vi "Demo - Generate Analog Out Data.vi"(9 "Phase Offset (Radians)":dbl[](array[numeric]), 10 "Number of Samples":i32, 11 "Number of AO Channels":i32) -> (3 "Sine Wave":i16[][](array[numeric]))   [LabVIEW 2017]
doc: "Generates a set of sine waves, with a phase offset."
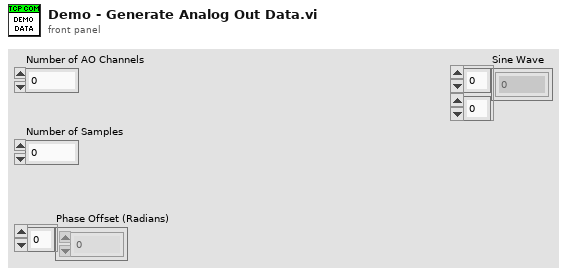
[diagram p1: front panel]
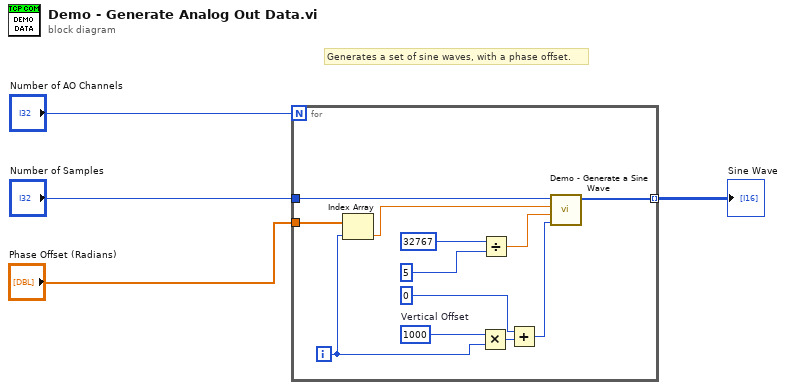
[diagram p0: block diagram]
diagram:
  # "Generates a set of sine waves, with a phase offset."
  n1 = for {
    N: "Number of AO Channels" -> [_]
    tunnel: "Number of Samples" -> [w13]
    tunnel: [w11] -> w4 mode=indexing
    tunnel: "Phase Offset (Radians)" -> [w10]
    i -> [w9]
    w12 = 1000  # Vertical Offset
    n2 = Index Array(array=w10, index=w9) -> (element=w8:dbl)
    n3 = Multiply(x=w12, y=w9) -> (x*y=w7:i32)
    n4 = Divide(x=i16 32767, y=5) -> (x/y=w14:dbl)
    n5 = Add(x=0, y=w7) -> (x+y=w5:i32)
    n6 = call "Demo - Generate a Sine Wave.vi"("Vertical Offset"=w5, "Peak Amplitude"=w14, "Phase Offset (Radians)"=w8, "Number of Samples"=w13) -> ("Sine Wave"=w11:i16[])  [unwired: 7 in]
  }
  "Sine Wave" <- w4
